vi "TRITON_REMOTE_Command.vi"(7 "Command to send":string, 8 "error in (no error)":errorcluster, 11 "IP Address":string="128.174.164.8") -> (0 "error out":errorcluster, 5 "Response String":string, 6 "Trimmed String":string)   [LabVIEW 2024]
panel:
  in  "Mode":T1(ring)=enum."Immediate"
  in  "Bytes to Read":i32=5000
  in  "Remote Port":i32=33576
  in  "Timeout":i32=10000
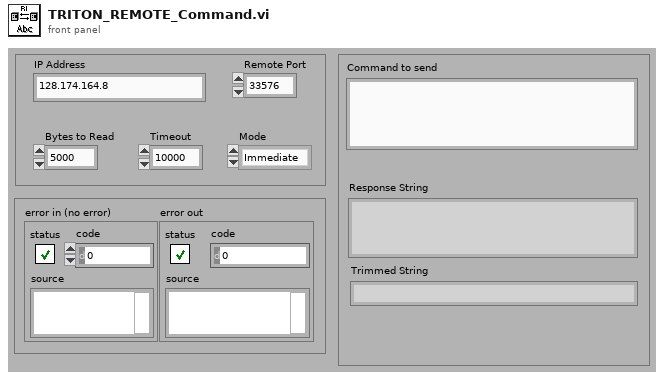
[diagram p1: front panel]
types:
  T1 = enum16{"Standard", "Buffered", "CRLF", "Immediate"}
  T2 = cluster{"Mode":enum16{"Standard", "Buffered", "CRLF", "Immediate"}, "Bytes to Read":i32, "IP Address":string, "Remote Port":i32, "Timeout":i32}
  T3 = cluster{"Mode":enum16{"Standard", "Buffered", "CRLF", "Immediate"}, "Bytes to Read":i32, "IP Address":string, "Remote Port":i32, "Timeout":i32, "connection ID":refnum<k5>}
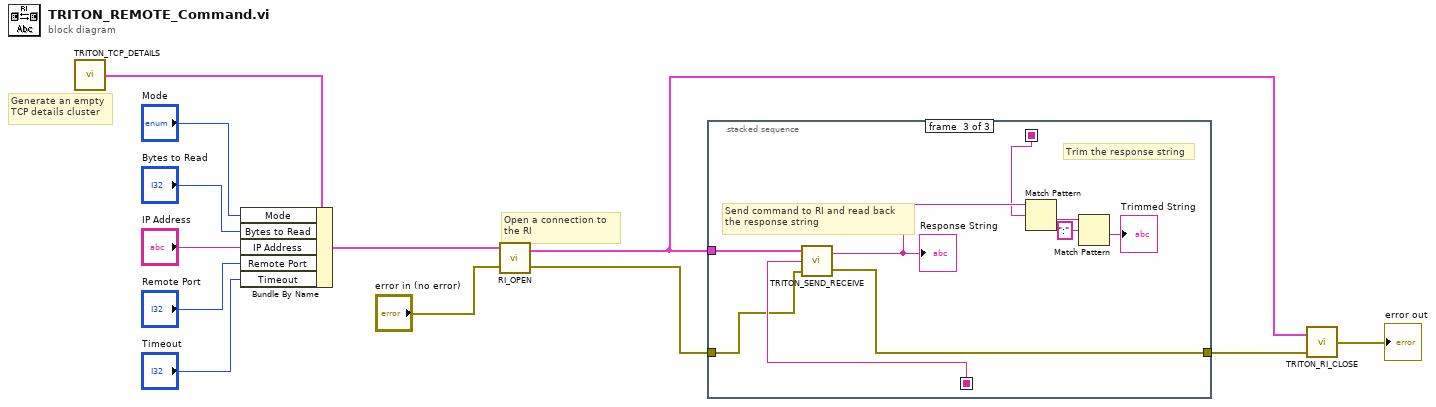
[diagram p0: block diagram]
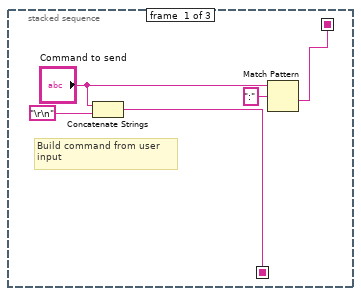
[diagram p2: hidden frame]
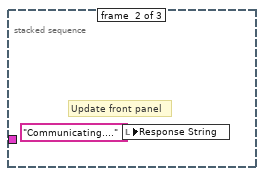
[diagram p3: hidden frame]
diagram:
  # "Open a connection to\nthe RI"
  # "Generate an empty\nTCP details cluster"
  n1 = call "TRITON_TCP_DETAILS.vi"() -> ("Cluster"=w12:T2)
  n2 = Bundle By Name(cluster=w12, "Mode"="Mode", "Bytes to Read"="Bytes to Read", "IP Address"="IP Address", "Remote Port"="Remote Port", "Timeout"="Timeout") -> (w10:T2)
  n3 = call "RI_OPEN.vi"("error in (no error)"="error in (no error)", "Cluster"=w10) -> ("error out"=w9:errorcluster, "output cluster"=w6:T3)
  n4 = stacked-sequence {
    seq-local: [w17 _ _] -> [_ _ w27]
    seq-local: [w14 _ _] -> [_ _ w23]
    tunnel: w9 -> [_ _ w26]
    tunnel: [_ _ w25] -> w8
    tunnel: w6 -> [_ _ w19]
    frame #0 {
      # "Build command from user\ninput"
      n5 = Concatenate Strings("Command to send", "\r\n") -> (w17:string)
      n6 = Match Pattern(string="Command to send", regular expression=":") -> (after substring=w14:string)  [unwired: 1 in, 3 out]
    }
    frame #1 {
      # "Update front panel"
      n7 = local write "Response String"("Communicating...." ("Response String")) -> ()
    }
    frame #2 {
      # "Trim the response string"
      # "Send command to RI and read back\nthe response string"
      n8 = call "TRITON_SEND_RECEIVE.vi"("error in (no error)"=w26, "Command String"=w27, "Communication Cluster"=w19) -> ("error out"=w25:errorcluster, "Response String"=w24:string)
      "Response String" <- w24
      n9 = Match Pattern(string=w24, regular expression=w23) -> (after substring=w22:string)  [unwired: 1 in, 3 out]
      n10 = Match Pattern(string=w22, regular expression=":") -> (after substring=→"Trimmed String":string)  [unwired: 1 in, 3 out]
    }
  }
  n11 = call "TRITON_RI_CLOSE.vi"("error in (no error)"=w8, "Communication Cluster"=w6) -> ("error out"=→"error out":errorcluster)
